vi "Untitled 3 (SubVI) 1.vi"(6 "select subPanel":bool, 9 "CtlRef":refnum<vi>, 10 "Boolean out":refnum<vi>, 11 "User Event in":refnum<user-event>) -> ()   [LabVIEW 2011]
uses:
  Controls/eventtypdef.ctl
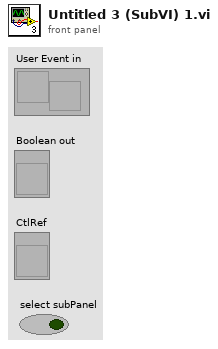
[diagram p1: front panel]
types:
  T1 = typedef "eventtypdef.ctl" = cluster{"label":string, "Sub Panel":refnum<vi>, "CtlRef":refnum<vi>, "This VI":refnum<vi>}
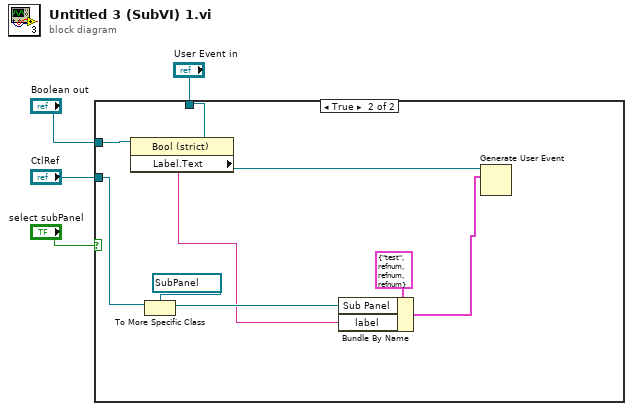
[diagram p0: block diagram]
diagram:
  n1 = case shown="True" "select subPanel" {
    tunnel: "User Event in" -> [_ w12]
    tunnel: "CtlRef" -> [_ w11]
    tunnel: "Boolean out" -> [_ w10]
    frame False {
    }
    frame True {
      n2 = property class="Bool (strict)"(reference=w10) -> ("Label.Text"=w5:string)  [unwired: 1 in, 2 out]
      n3 = To More Specific Class(target class=refnum<vi> refnum ("Sub Panel"), reference=w11) -> (specific class reference=w7:refnum<vi>)  [unwired: 1 in, 1 out]
      n4 = Bundle By Name(cluster=T1 {"label"="test", "Sub Panel"=refnum, "CtlRef"=refnum, "This VI"=refnum} ("event data"), "Sub Panel"=w7, "label"=w5) -> (w6:T1)
      n5 = Generate User Event(user event=w12, event data cluster=w6) -> ()  [unwired: 1 in, 2 out]
    }
  }
